vi "HolographySimulation.vi"() -> ()   [LabVIEW 2015]
panel:
  in  "Exposure":dbl
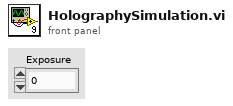
[diagram p1: front panel]
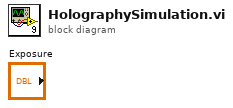
[diagram p0: block diagram]
diagram:
